vi "niRFUtil MT Apply IQ Impairments.vi"(0 "Waveform In":T1={"x0"=0.0, "dx"=1.0, "y"=[]} caption="input complex waveform" {"y" format="%.2f"; "dx" format="%^.2e"; "x0" format="%^.2e"}, 1 "I DC offset (%)":dbl format="%.2f", 2 "impairment definition":enum16{"Vertical Shear", "Axis Shear"}(ring), 5 "Q DC offset (%)":dbl format="%.2f", 7 "IQ gain imbalance (dB)":dbl format="%.2f", 9 "quadrature skew (deg)":dbl format="%.2f", 11 "error in (no error)":errorcluster, 12 "frequency offset (Hz)":dbl format="%.2f", 13 "reset? (T)":bool=TRUE) -> (4 "Waveform Out":T1 caption="output complex waveform" {"y" format="%.2f"; "dx" format="%^.2e"; "x0" format="%^.2e"}, 15 "error out":errorcluster)   [LabVIEW 2015, in "niRFUtil.lvlib"]
doc: "Applies various I/Q impairments to the complex baseband modulated waveform."
uses:
  niRFUtil.lvlib
  Includes/niRFUtil INC Complex Waveform.ctl
  Includes/niRFUtil INC Complex Array.ctl
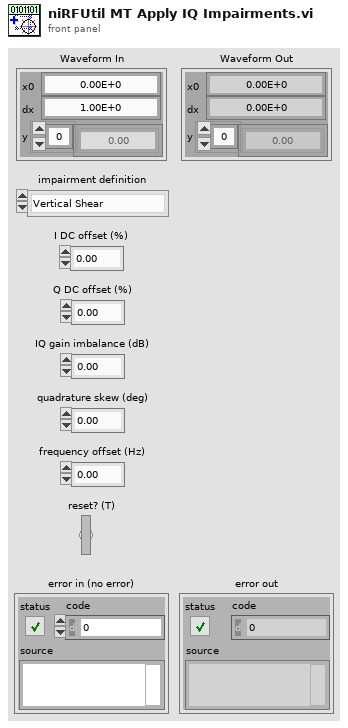
[diagram p1: front panel]
types:
  T1 = typedef "niRFUtil.lvlib/niRFUtil INC Complex Waveform.ctl" = cluster{"x0":dbl, "dx":dbl, "y":T2}
  T2 = typedef "niRFUtil.lvlib/niRFUtil INC Complex Array.ctl" = csg[]
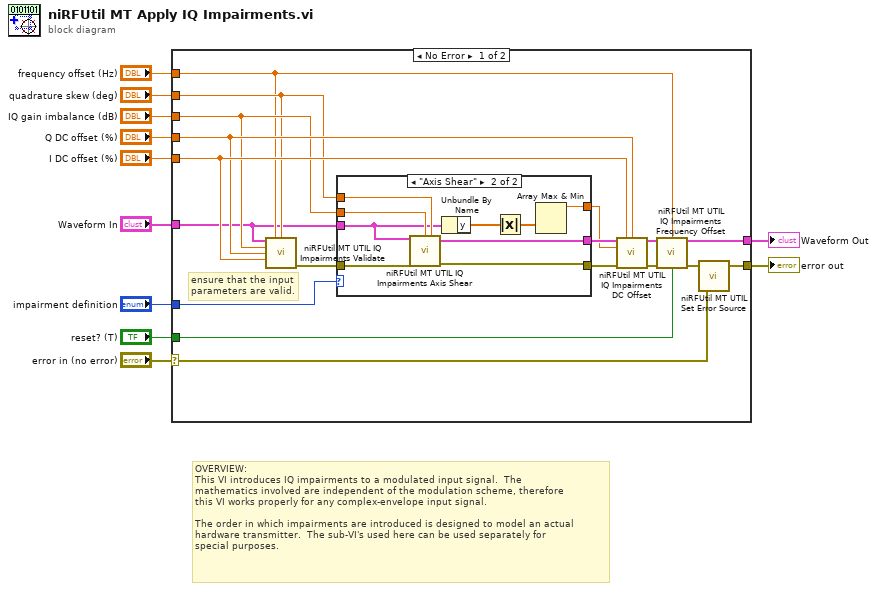
[diagram p0: block diagram]
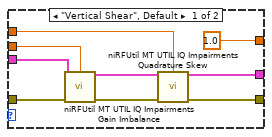
[diagram p2: hidden frame]
diagram:
  # "OVERVIEW:\nThis VI introduces IQ impairments to a modulated input signal.  The\nmathematics involved are independent of the modulation scheme, therefore\nthis VI works properly for any complex-envelope input signal.\n\nThe order in which impairments are introduced is designed to model an actual\nhardware transmitter.  The sub-VI's used here can be used separately for\nspecial purposes."
  n1 = case shown="No Error" "error in (no error)" {
    selector: "error in (no error)" -> [w19 w48]
    tunnel: "reset? (T)" -> [w29 _]
    tunnel: [w21 w48] -> w9
    tunnel: [w25 w49] -> w8
    tunnel: "Waveform In" -> [w13 w49]
    tunnel: "I DC offset (%)" -> [w28 _]
    tunnel: "Q DC offset (%)" -> [w27 _]
    tunnel: "IQ gain imbalance (dB)" -> [w26 _]
    tunnel: "quadrature skew (deg)" -> [w24 _]
    tunnel: "frequency offset (Hz)" -> [w15 _]
    tunnel: "impairment definition" -> [w14 _]
    frame No Error {
      # "ensure that the input parameters are valid."
      n2 = call "niRFUtil MT UTIL IQ Impairments Validate.vi"("Waveform In"=w13, "frequency offset (Hz)"=w15, "Quadrature Skew, deg"=w24, "IQ Gain Imbalance, dB"=w26, "Q DC Offset, %"=w27, "I DC Offset, %"=w28) -> ("error out"=w16:errorcluster)  [unwired: 9 out]
      n3 = case shown="\"Axis Shear\"" w14 {
        tunnel: w26 -> [w38 w44]
        tunnel: w24 -> [w37 w43]
        tunnel: w13 -> [w36 w42]
        tunnel: [w34 w45] -> w18
        tunnel: [w33 w46] -> w17
        tunnel: w16 -> [w31 w47]
        tunnel: [1.0 w39] -> w12
        frame "Vertical Shear", Default {
          n4 = call "niRFUtil MT UTIL IQ Impairments Gain Imbalance.vi"("Waveform In"=w36, "IQ Gain Imbalance, dB"=w38, "error in (no error)"=w31) -> ("Waveform Out"=w35:T1, "error out"=w32:errorcluster)  [unwired: 11 out]
          n5 = call "niRFUtil MT UTIL IQ Impairments Quadrature Skew.vi"("Waveform In"=w35, "Quadrature Skew, deg"=w37, "error in (no error)"=w32) -> ("Waveform Out"=w34:T1, "error out"=w33:errorcluster)  [unwired: 11 out]
        }
        frame "Axis Shear" {
          n6 = call "niRFUtil MT UTIL IQ Impairments Axis Shear.vi"("Waveform In"=w42, "IQ Gain Imbalance, dB"=w44, "Quadrature Skew, degrees"=w43, "error in (no error)"=w47) -> ("Waveform Out"=w45:T1, "error out"=w46:errorcluster)  [unwired: 10 out]
          n7 = Unbundle By Name(w42) -> ("y"=w40:T2)
          n8 = Absolute Value(x=w40) -> (abs(x)=w41:sgl[])
          n9 = Array Max & Min(array=w41) -> (max value=w39:sgl)  [unwired: 3 out]
        }
      }
      n10 = call "niRFUtil MT UTIL IQ Impairments DC Offset.vi"("Waveform In"=w18, "I DC Offset, %"=w28, "Q DC Offset, %"=w27, "Gain Scaling factor"=w12, "error in (no error)"=w17) -> ("Waveform Out"=w22:T1, "error out"=w23:errorcluster)  [unwired: 9 out]
      n11 = call "niRFUtil MT UTIL IQ Impairments Frequency Offset.vi"("Waveform In"=w22, "Frequency Offset, Hz"=w15, "error in (no error)"=w23, "Reset? (T)"=w29) -> ("Waveform Out"=w25:T1, "error out"=w20:errorcluster)  [unwired: 10 out]
      n12 = call "niRFUtil MT UTIL Set Error Source.vi"("initial error in (no error)"=w19, "final error in (no error)"=w20) -> ("error out"=w21:errorcluster)  [unwired: 3 in]
    }
    frame Error {
    }
  }
  "error out" <- w9
  "Waveform Out" <- w8
